vi "Value Handler.vi"(10 "Set or Get":enum16{"Set", "Get"}(ring), 11 "PID gains":T1={"proportional gain (Kc)"=0.0111, "integral time (Ti, min)"=0.007, "derivative time (Td, min)"=0.0}) -> (3 "PID gains Out":T1={"proportional gain (Kc)"=0.0111, "integral time (Ti, min)"=0.007, "derivative time (Td, min)"=0.0})   [LabVIEW 2011, in "Pivot Drive.lvlib"]
uses:
  Pivot Drive.lvlib
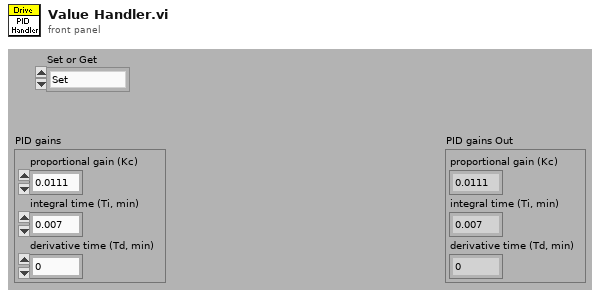
[diagram p1: front panel]
types:
  T1 = cluster{"proportional gain (Kc)":dbl, "integral time (Ti, min)":dbl, "derivative time (Td, min)":dbl}
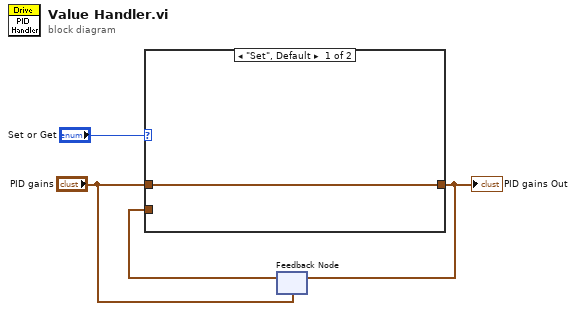
[diagram p0: block diagram]
diagram:
  n1 = feedback #1("PID gains") -> (w2:T1)
  n2 = case shown="\"Set\", Default" "Set or Get" {
    tunnel: "PID gains" -> [w5 _]
    tunnel: [w5 w6] -> w3
    tunnel: w2 -> [_ w6]
    frame "Set", Default {
    }
    frame "Get" {
    }
  }
  "PID gains Out" <- w3
  n3 = feedback-in #1(w3) -> ()
